vi "Write.vi"(8 "error in (no error)":errorcluster, 9 "write enable":bool=TRUE, 11 "ICPCON ET7042 in":refnum<class "ICPCON ET-7042.lvclass">) -> (0 "error out":errorcluster, 3 "ICPCON ET7042 out":refnum<class "ICPCON ET-7042.lvclass">)   [LabVIEW 2021, in "ICPCON ET-7042.lvclass"]
uses:
  ICPCON ET-7042.lvclass
  D:/my_projects/projects/21/Master CR/Master CR.lvclass
  D:/my_projects/projects/21/Master CR/Devices/ET7000/TCP/TCP.lvclass
  Master CR.lvclass/Master CR.ctl
  Modbus_v121c/Modbus Data Unit/Modbus Data Unit.lvclass/Modbus Data Unit.ctl
  Modbus_v121c/Network Protocol/Network Master/Network Master.lvclass/Network Master.ctl
  Modbus_v121c/Master Function Definition/Write Multiple Coils Request.vi
  Modbus_v121c/Master Function Definition/Function data mismatch error.vi
  Modbus_v121c/Master Function Definition/Write Multiple Coils Response.vi
  Modbus_v121c/Network Protocol/Network Master/Read write Master.vi
  Network Protocol/Read Network Protocol.vi
  Modbus_v121c/Modbus Data Unit/Construct PDU.vi
  Modbus_v121c/Utility/Bits to Bytes.vi
  Modbus_v121c/Data Model/Error Generator.vi
  Modbus_v121c/Master Function Definition/Function code mismatch error.vi
  Modbus_v121c/Modbus Data Unit/Deconstruct PDU.vi
  TCP/TCP.lvclass
  Modbus_v121c/Network Protocol/Network Master/Network Master.lvclass
  Modbus_v121c/Modbus Data Unit/Modbus Data Unit.lvclass
  Modbus_v121c/Data Model/Device Data Model.lvclass
  Modbus_v121c/Transmission Data Unit/Transmission Data Unit.lvclass
  Master CR.lvclass
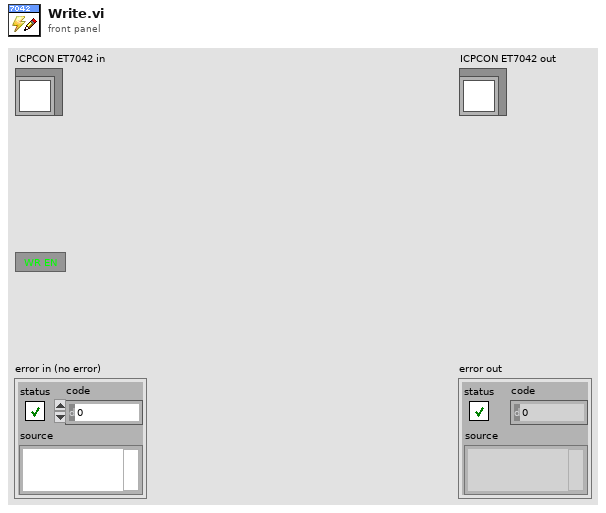
[diagram p1: front panel]
types:
  T1 = typedef "Device Data Model.lvclass/N channel.ctl" = cluster{"N DI channel":i32, "N DO channel":i32, "N AI channel":i32, "N AO channel":i32}
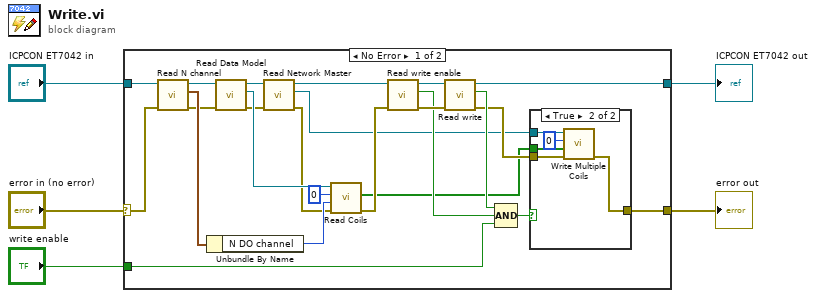
[diagram p0: block diagram]
diagram:
  n1 = case shown="No Error" "error in (no error)" {
    selector: "error in (no error)" -> [w26 w37]
    tunnel: [w17 w37] -> w3
    tunnel: [w9 w36] -> w4
    tunnel: "ICPCON ET7042 in" -> [w28 w36]
    tunnel: "write enable" -> [w8 _]
    frame No Error {
      n2 = call "Read N channel.vi"("error in (no error)"=w26, "Master CR in"=w28) -> ("error out"=w25:errorcluster, "N channel"=w29:T1, "Master CR out"=w27:refnum<class "ICPCON ET-7042.lvclass">)  [unwired: 7 in]
      n3 = Unbundle By Name(w29) -> ("N DO channel"=w19:i32)
      n4 = call "Read Data Model.vi"("error in (no error)"=w25, "Master CR in"=w27) -> ("error out"=w11:errorcluster, "Data Model"=w16:refnum<class "Device Data Model.lvclass">, "Master CR out"=w12:refnum<class "ICPCON ET-7042.lvclass">)  [unwired: 7 in]
      n5 = call "Read Network Master.vi"("error in (no error)"=w11, "TCP in"=w12) -> ("error out"=w7:errorcluster, "Network Master"=w6:refnum<class "Network Master.lvclass">, "TCP out"=w10:refnum<class "ICPCON ET-7042.lvclass">)  [unwired: 7 in]
      n6 = call-dynamic "Read Coils.vi"("error in"=w7, "number of coils"=w19, "starting address"=u16 0, "device data model in"=w16) -> ("error out"=w15:errorcluster, "data"=w13:bool[])  [unwired: 5 in, 1 out]
      n7 = call "Read write enable.vi"("error in (no error)"=w15, "Master CR in"=w10) -> ("error out"=w23:errorcluster, "write enable"=w20:bool, "Master CR out"=w24:refnum<class "ICPCON ET-7042.lvclass">)  [unwired: 7 in]
      n8 = call "Read write.vi"("error in (no error)"=w23, "Master CR in"=w24) -> ("error out"=w14:errorcluster, "Write"=w21:bool, "Master CR out"=w9:refnum<class "ICPCON ET-7042.lvclass">)  [unwired: 7 in]
      n9 = Compound Arithmetic op=AND(w21, w20, w8) -> (w22:bool)
      n10 = case shown="True" w22 {
        tunnel: w14 -> [w30 w35]
        tunnel: [w30 w32] -> w17
        tunnel: w13 -> [_ w34]
        tunnel: w6 -> [_ w31]
        frame False {
        }
        frame True {
          n11 = call "Write Multiple Coils.vi"("error in (no error)"=w35, "coil values"=w34, "starting address"=u16 0, "Modbus master in"=w31) -> ("error out"=w32:errorcluster)  [unwired: 6 in, 1 out]
        }
      }
    }
    frame Error {
    }
  }
  "error out" <- w3
  "ICPCON ET7042 out" <- w4
